vi "Open Device.vi"(8 "error in (no error)":errorcluster, 11 "Device in":refnum<class "Device.lvclass">) -> (0 "error out":errorcluster, 3 "Device out":refnum<class "Device.lvclass">)   [LabVIEW 2012, in "HAL.lvlib" / "Device.lvclass"]
doc: "Opening a device corresponds to getting the device ready to interact with. This may involve opening a serial port, GPIB bus, ethernet connection, or some other means of interacting with the device. If there is a problem getting the device ready to interact with then this VI should return an appropriate error. This VI should perform some action to verify communication with the device, such as checking a device ID, name, or version so that the chance of issues occurring later are reduced."
uses:
  Device.lvclass
  <vilib>/Utility/error.llb/Error Cluster From Error Code.vi
  <vilib>/ErrorRing/Error Ring.xnode
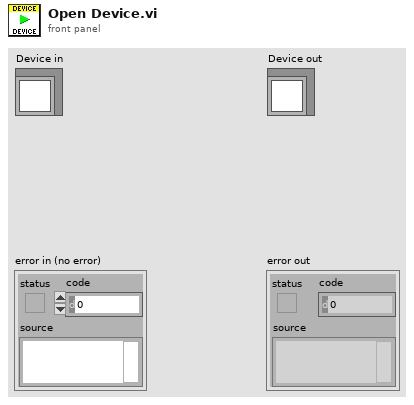
[diagram p1: front panel]
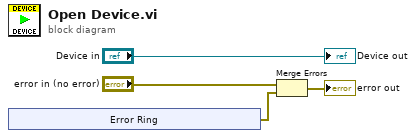
[diagram p0: block diagram]
diagram:
  n1 = xnode "Error Ring"() -> ("error out"=w3:errorcluster)
  n2 = Merge Errors("error in (no error)", w3) -> (→"error out":errorcluster)
  "Device out" <- "Device in"
